vi "Data Logging TDMS DAQ.vi"() -> ()   [LabVIEW 2020]
panel:
  out "Waveform Graph":dynamicdata(graph)
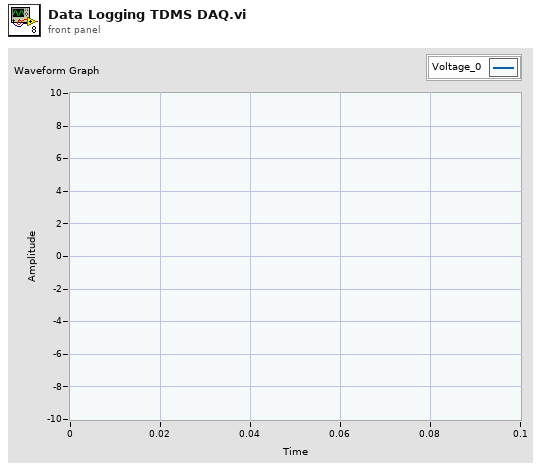
[diagram p1: front panel]
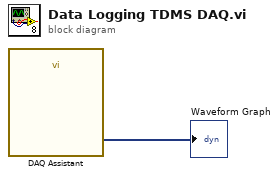
[diagram p0: block diagram]
diagram:
  n1 = call "DAQ Assistant"() -> ("data"=→"Waveform Graph":dynamicdata)  [unwired: 17 in, 2 out]
